vi "VG_OFF.vi"() -> ()   [LabVIEW 2020]
panel:
  out "OFF":bool
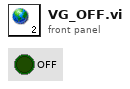
[diagram p1: front panel]
diagram:
